vi "Adjustable Filter.vi"(7 "Filter Type":T1, 9 "Reset Filter":bool, 10 "Frequency":dbl, 11 "Audio Data":dbl[](array[numeric])) -> (3 "Filtered Audio Data":dbl[](array[numeric]))   [LabVIEW 2018, in "Channel.lvclass"]
uses:
  Channel.lvclass
  <vilib>/Analysis/3filter.llb/Filter Passband Type.ctl
  Libraries/Globals/Constants.vi
  <vilib>/Analysis/3filter.llb/Bessel Filter (DBL).vi
  <vilib>/Analysis/NI_AALBase.lvlib
  Libraries/Globals/Globals.lvlib
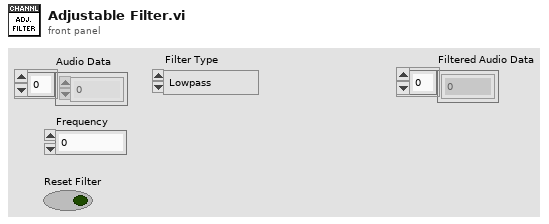
[diagram p1: front panel]
types:
  T1 = typedef "NI_AALBase.lvlib/Filter Passband Type.ctl" = enum32{"Lowpass", "Highpass", "Bandpass", "Bandstop"}
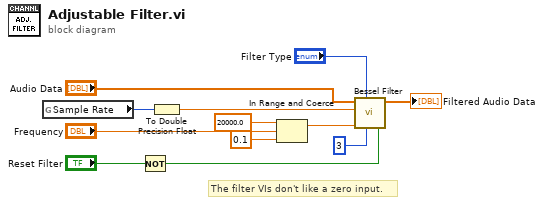
[diagram p0: block diagram]
diagram:
  # "The filter VIs don't like a zero input."
  n1 = global read "Constants.vi" "Sample Rate"() -> (w5:i32)
  n2 = Not(x="Reset Filter") -> (.not. x?=w1:bool)
  n3 = To Double Precision Float(number=w5) -> (double precision float=w4:dbl)
  n4 = In Range and Coerce(upper limit=20000.0 ("y"), x="Frequency", lower limit=0.1) -> (coerced(x)=w8:dbl)  [unwired: 1 out]
  n5 = call-poly <vilib>:"Bessel Filter.vi"("init/cont (init:F)"=w1, "order"=3, "filter type"="Filter Type", "low cutoff freq: fl"=w8, "sampling freq: fs"=w4, "X"="Audio Data") -> ("Filtered X"=→"Filtered Audio Data":dbl[])  [unwired: 2 in, 1 out]
